vi "ActiveObject_QueueQueue_StopProcess.vi"(0 "reference in":refnum<class>, 2 "ms timeout (-1)":i32=-1, 5 "error in (no error)":errorcluster) -> (14 "reference out":refnum<class>, 19 "error out":errorcluster)   [LabVIEW 2012]
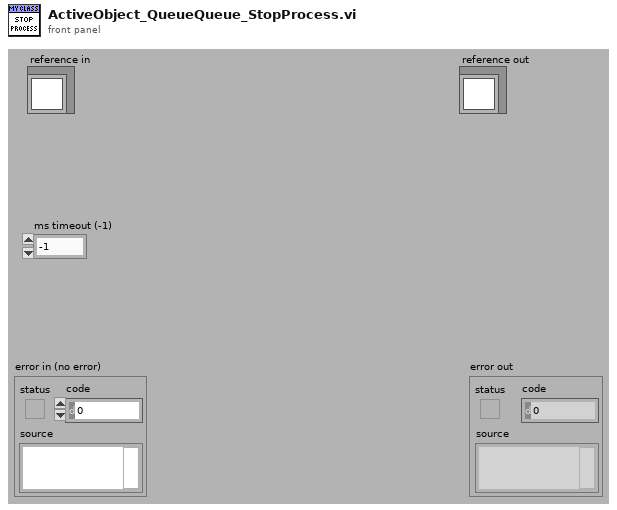
[diagram p1: front panel]
types:
  T1 = enum16{"ReadRepository", "CreateNew", "CreateOrLookUpExisting", "ReadRepositoryAndDestroy"}
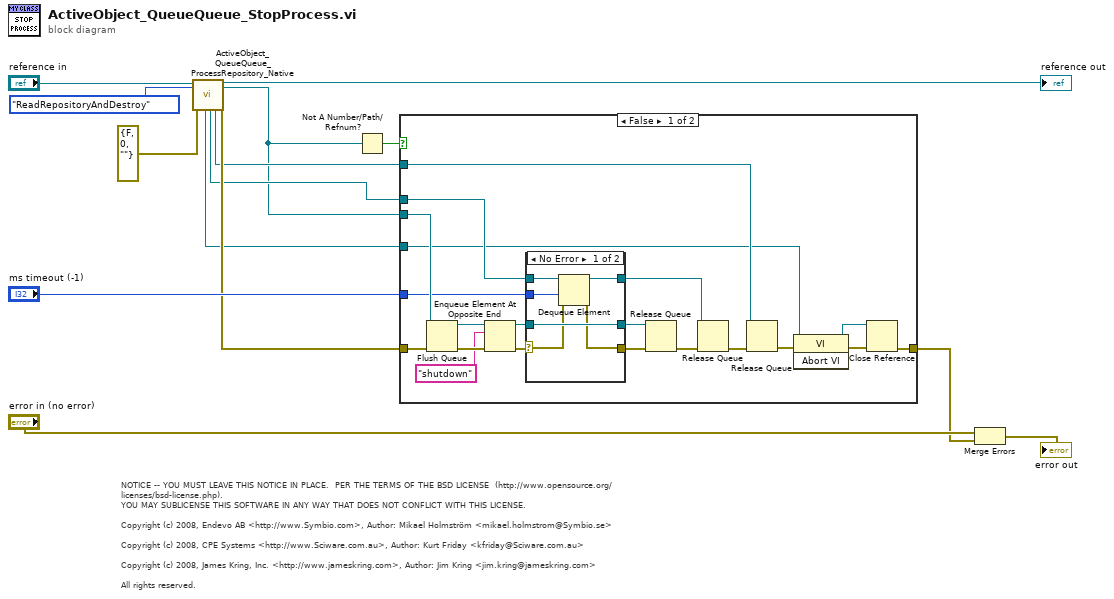
[diagram p0: block diagram]
diagram:
  # "NOTICE -- YOU MUST LEAVE THIS NOTICE IN PLACE.  PER THE TERMS OF THE BSD LICENSE  (http://www.opensource.org/licenses/bsd-license.php).\nYOU MAY SUBLICENSE THIS SOFTWARE IN ANY WAY THAT DOES NOT CONFLICT WITH THIS LICENSE.\n\nCopyright (c) 2008, Endevo AB <http://www.Symbio.com>, Author: Mikael Holmström <mikael.holmstrom@Symbio.se>\n\nCopyright (c) 2008, CPE Systems <http://www.Sciware.com.au>, Author: Kurt Friday <kfriday@Sciware.com.au>\n\nCopyright (c) 2008, James Kring, Inc. <http://www.jameskring.com>, Author: Jim Kring <jim.kring@jameskring.com>\n\nAll rights reserved."
  n1 = call <resource>:"ActiveObject_QueueQueue_ProcessRepository_Native.vi"("reference in"="reference in", "Action(ReadRepository)"=T1."ReadRepositoryAndDestroy", "error in (no error)"=errorcluster {"status"=FALSE, "code"=0, "source"=""}) -> ("ProcessViRef"=w5:refnum<vi>, "ProcessSyncQueue"=w7:refnum<queue>, "FromProcessQueue"=w6:refnum<queue>, "reference out"=→"reference out":refnum<class>, "ToProcessQueue"=w3:refnum<queue>, "error out"=w8:errorcluster)  [unwired: 10 in, 1 out]
  n2 = Not A Number/Path/Refnum?(number/path/refnum=w3) -> (NaN/Path/Refnum?=w2:bool)
  n3 = case shown="False" w2 {
    tunnel: w7 -> [w29 _]
    tunnel: w8 -> [w31 w44]
    tunnel: [w25 w44] -> w12
    tunnel: w3 -> [w34 _]
    tunnel: "ms timeout (-1)" -> [w24 _]
    tunnel: w6 -> [w22 _]
    tunnel: w5 -> [w16 _]
    frame False {
      n4 = Flush Queue(queue=w34, error in (no error)=w31) -> (queue out=w32:refnum<queue>, error out=w33:errorcluster)  [unwired: 1 out]
      n5 = Enqueue Element At Opposite End(queue=w32, element="shutdown", error in (no error)=w33) -> (queue out=w28:refnum<queue>, error out=w23:errorcluster)  [unwired: 1 in, 1 out]
      n6 = case shown="No Error" w23 {
        tunnel: [w36 w43] -> w27
        tunnel: w29 -> [w39 w41]
        tunnel: [w40 w42] -> w26
        tunnel: w28 -> [w40 w42]
        tunnel: w24 -> [w38 _]
        selector: w23 -> [w37 w43]
        tunnel: [w35 w41] -> w20
        frame No Error {
          n7 = Dequeue Element(queue=w39, timeout in ms (-1)=w38, error in (no error)=w37) -> (queue out=w35:refnum<queue>, error out=w36:errorcluster)  [unwired: 2 out]
        }
        frame Error {
        }
      }
      n8 = Release Queue(queue=w26, error in (no error)=w27) -> (error out=w21:errorcluster)  [unwired: 1 in, 2 out]
      n9 = Release Queue(queue=w20, error in (no error)=w21) -> (error out=w19:errorcluster)  [unwired: 1 in, 2 out]
      n10 = Release Queue(queue=w22, error in (no error)=w19) -> (error out=w18:errorcluster)  [unwired: 1 in, 2 out]
      n11 = invoke class="VI" method="Abort VI"(reference=w16, error in=w18) -> (reference out=w15:refnum<vi>, error out=w17:errorcluster)  [unwired: 1 in, 1 out]
      n12 = Close Reference(reference=w15, error in (no error)=w17) -> (error out=w25:errorcluster)
    }
    frame True {
    }
  }
  n13 = Merge Errors("error in (no error)", w12) -> (→"error out":errorcluster)
